vi "引用測試.vi"() -> ()   [LabVIEW 2015]
uses:
  <vilib>/vision/Measure.llb/Edge Options.ctl
  <vilib>/vision/Measure.llb/Edge Polarity.ctl
  <vilib>/vision/NI_Vision_Development_Module.lvlib
panel:
  in  "Gap 2":i32=10 min=1 max=300
  in  "Edge Options 2":T1={"Edge Polarity"=0, "Kernel Size"=3, "Width"=3, "Minimum Edge Strength"=10.0, "Interpolation Type"=enum."Bilinear Fixed", "Data Processing Method"=enum."Average"} {"Edge Polarity" items=["All Edges", "Rising Edges", "Falling Edges"]; "Minimum Edge Strength" format="%.2f"; "Width" step=2; "Kernel Size" step=2}
  in  "Process 2":T3(ring)
  in  "Process":T3(ring)
  out "Line Profile":T4(graph)
  in  "Edge Options":T1={"Edge Polarity"=0, "Kernel Size"=3, "Width"=3, "Minimum Edge Strength"=10.0, "Interpolation Type"=enum."Bilinear Fixed", "Data Processing Method"=enum."Average"} {"Edge Polarity" items=["All Edges", "Rising Edges", "Falling Edges"]; "Minimum Edge Strength" format="%.2f"; "Width" step=2; "Kernel Size" step=2}
  out "Gradient Information":dbl[][](graph)
  out "error out 2":errorcluster
  out "Ellipse":T5 {"Minor Axis"."Point 2"."Y" format="%.2f"; "Minor Axis"."Point 2"."X" format="%.2f"; "Minor Axis"."Point 1"."Y" format="%.2f"; "Minor Axis"."Point 1"."X" format="%.2f"; "Major Axis"."Point 2"."Y" format="%.2f"; "Major Axis"."Point 2"."X" format="%.2f"; "Major Axis"."Point 1"."Y" format="%.2f"; "Major Axis"."Point 1"."X" format="%.2f"; "Center"."Y" format="%.2f"; "Center"."X" format="%.2f"}
  out "x-y":u32
  out "error out":errorcluster
  in  "Direction 2":T6(ring)
  in  "Direction":enum16{"Inner to Outer", "Outer to Inner"}(ring)
  in  "ROI":T7
  in  "Gap":i32=10 min=1 max=300
  out "Image":T8(plugin-control)
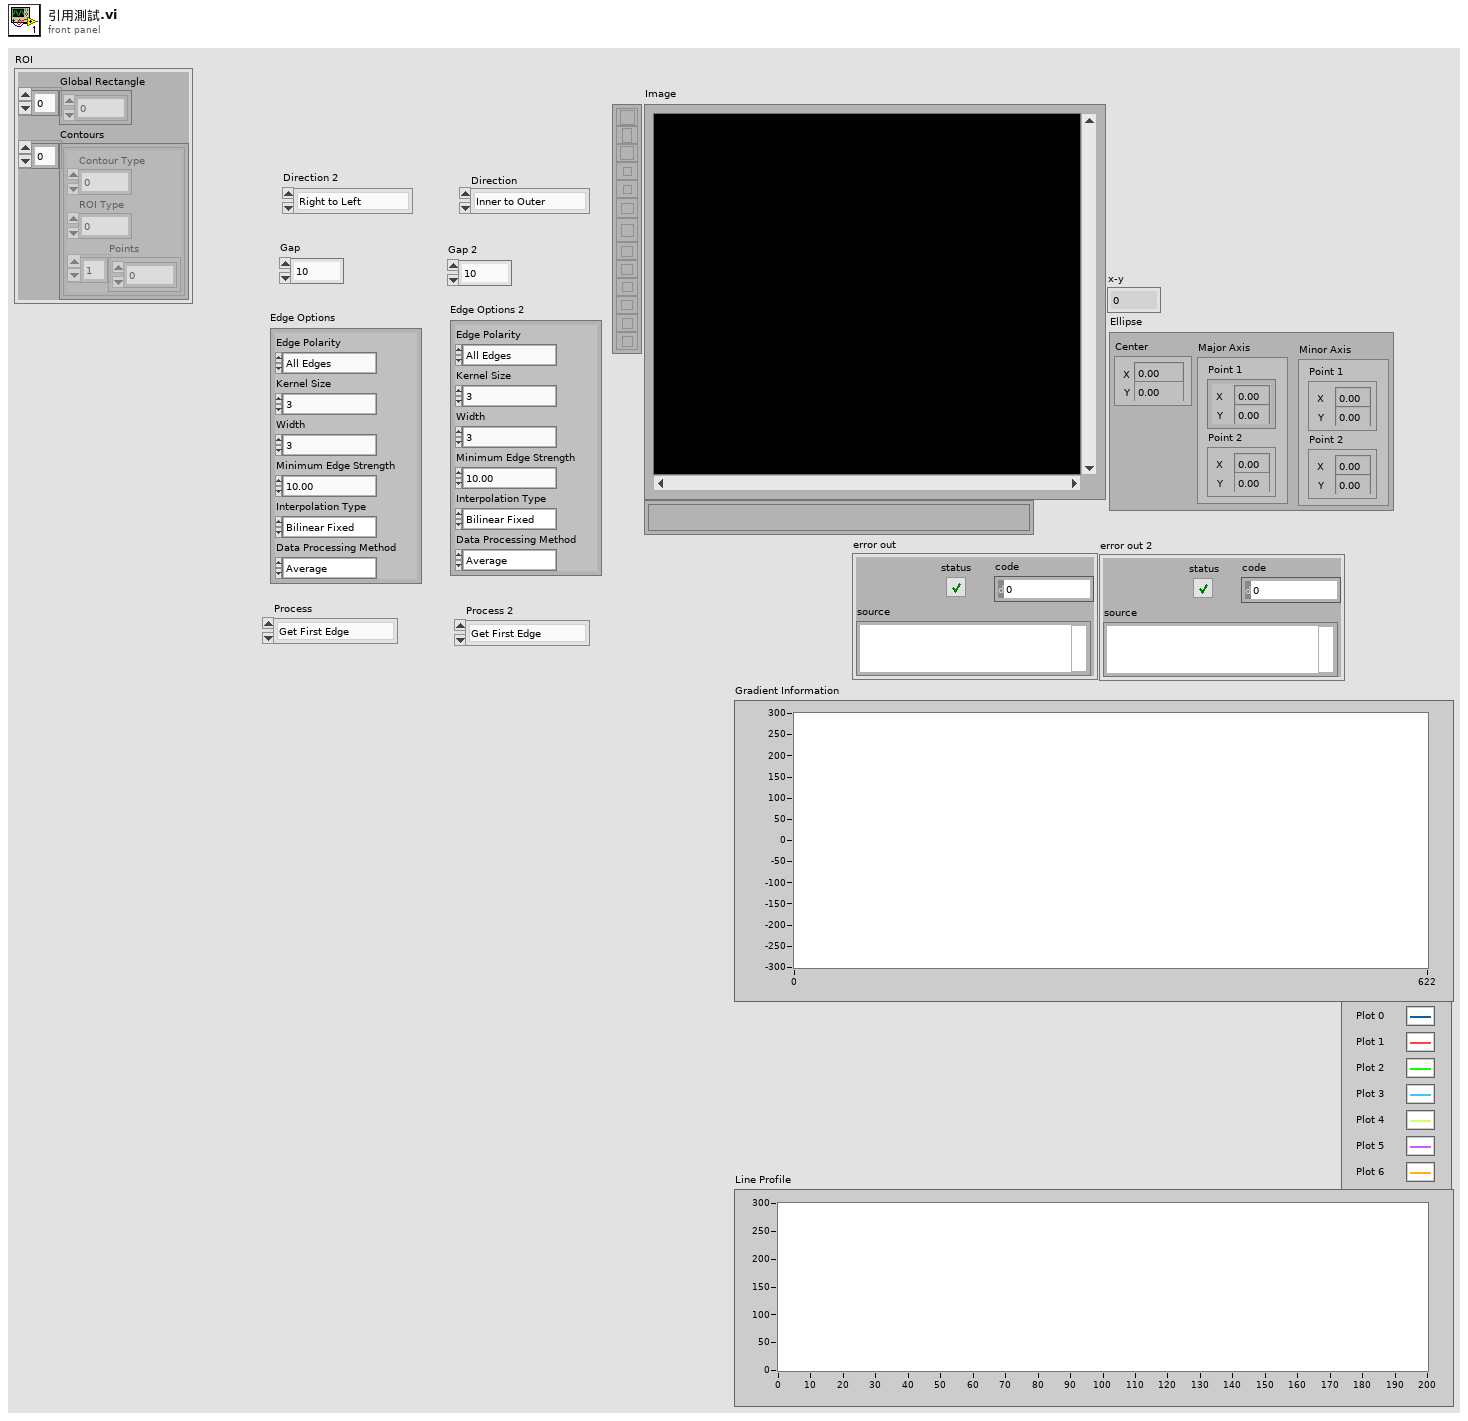
[diagram p1: front panel]
types:
  T1 = typedef "Edge Options.ctl" = cluster{"Edge Polarity":T2, "Kernel Size":u32, "Width":u32, "Minimum Edge Strength":sgl, "Interpolation Type":enum32{"Zero Order", "Bilinear", "Quadratic", "Cubic", "Bilinear Fixed"}, "Data Processing Method":enum32{"Average", "Median"}}
  T2 = typedef "Edge Polarity.ctl" = u32
  T3 = enum16{"Get First Edge", "Get First + Last Edge", "Get All Edges", "Get Best Edge"}
  T4 = cluster{"x0":sgl, "dx":sgl, "Pixels Line":sgl[]}[]
  T5 = cluster{"Center":cluster{"X":sgl, "Y":sgl}, "Major Axis":cluster{"Point 1":cluster{"X":sgl, "Y":sgl}, "Point 2":cluster{"X":sgl, "Y":sgl}}, "Minor Axis":cluster{"Point 1":cluster{"X":sgl, "Y":sgl}, "Point 2":cluster{"X":sgl, "Y":sgl}}}
  T6 = enum16{"Right to Left", "Left  to Right", "Up to Down", "Down to Up"}
  T7 = cluster{"Global Rectangle":i32[], "Contours":cluster{"Contour Type":u32, "ROI Type":u32, "Points":i32[]}[]}
  T8 = typedef "IMAQ Image.ctl" = refnum<image>
  T9 = typedef "Image Type" = u32
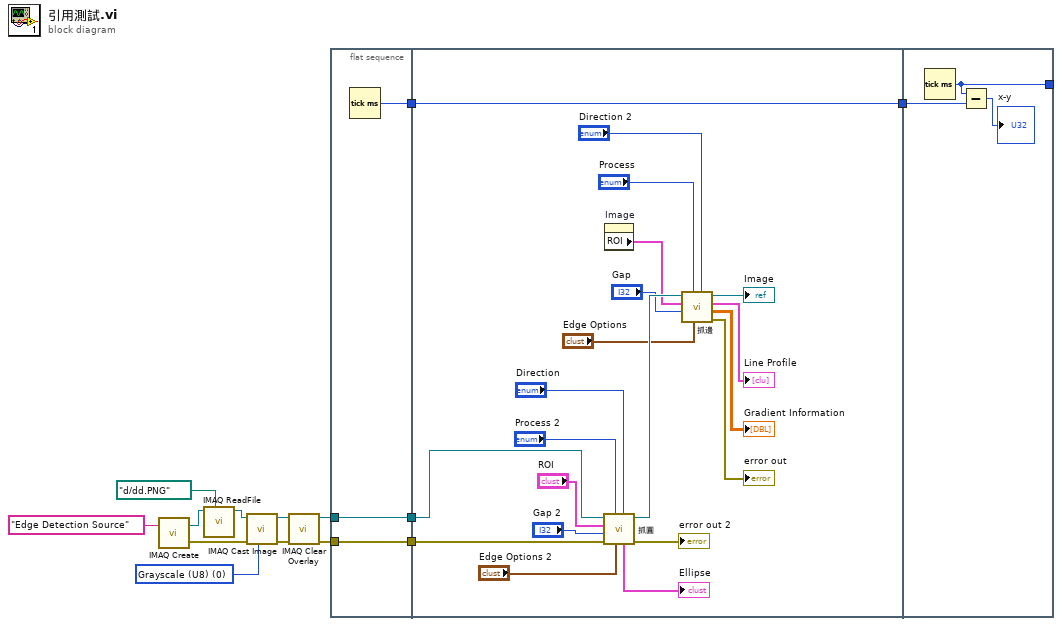
[diagram p0: block diagram]
diagram:
  w13 = T9 0 items=["Grayscale (U8)", "Grayscale (I16)", "Grayscale (SGL)", "Complex (CSG)", "RGB (U32)", "HSL (U32)", "RGB (U64)", "Grayscale (U16)"] ("Image Type")
  n1 = call "IMAQ Create"("Image Name"="Edge Detection Source") -> ("New Image"=w11:T8, "error out"=w12:errorcluster)  [unwired: 4 in]
  n2 = call "IMAQ ReadFile"("File Path"=path "d:/dd.PNG", "Image"=w11) -> ("Image Out"=w10:T8)  [unwired: 5 in, 4 out]
  n3 = call "IMAQ Cast Image"("Image Type"=w13, "error in (no error)"=w12, "Image Src"=w10) -> ("error out"=w6:errorcluster, "Image Dst Out"=w9:T8)  [unwired: 7 in]
  n4 = call "IMAQ Clear Overlay"("error in (no error)"=w6, "Image"=w9) -> ("error out"=w7:errorcluster, "Image Out"=w8:T8)  [unwired: 8 in]
  n5 = flat-sequence {
    tunnel: w7 -> [w16]
    tunnel: w8 -> [w17]
    tunnel: [w17] -> w5
    tunnel: [w16] -> w4
    tunnel: [w15] -> w3
    tunnel: w5 -> [w31]
    tunnel: w4 -> [w30]
    tunnel: w3 -> [w28]
    tunnel: [w28] -> w2
    tunnel: [w40] -> _
    tunnel: w2 -> [w39]
    frame #0 {
      n6 = Tick Count (ms)() -> (millisecond timer value=w15:u32)
    }
    frame #1 {
      n7 = call "抓圓.vi"("Direction"="Direction", "Edge Options"="Edge Options 2", "Process"="Process 2", "error In"=w30, "Gap"="Gap 2", "ROI"="ROI", "Image In"=w31) -> ("error out"=→"error out 2":errorcluster, "Image"=w35:T8, "Ellipse"=→"Ellipse":T5)  [unwired: 2 out]
      n8 = property on="Image" class="ImageControl"() -> ("ROI"=w22:T7)  [unwired: 2 in, 2 out]
      n9 = call "抓邊.vi"("Direction"="Direction 2", "Edge Options"="Edge Options", "Process"="Process", "Gap"="Gap", "ROI"=w22, "Image In"=w35) -> ("error out"=→"error out":errorcluster, "Gradient Information"=→"Gradient Information":dbl[][], "Line Profile"=→"Line Profile":T4, "Image"=→"Image":T8)  [unwired: 1 in, 1 out]
    }
    frame #2 {
      n10 = Tick Count (ms)() -> (millisecond timer value=w40:u32)
      n11 = Subtract(x=w40, y=w39) -> (x-y=→"x-y":u32)
    }
  }
